vi "RX ADU.vi"(8 "error in (no error)":errorcluster, 9 "PDU_req":T1={"Function Code"=1, "Data"=[], "RTU_DataBytes"=0}, 10 "TCP connection in":refnum<k5>, 11 "MB_ADU_TCP in":refnum<class "MB_ADU_TCP.lvclass">) -> (0 "error out":errorcluster, 1 "PDU_resp":T1={"Function Code"=1, "Data"=[], "RTU_DataBytes"=0}, 2 "TCP connection out":refnum<k5>, 3 "MB_ADU_TCP out":refnum<class "MB_ADU_TCP.lvclass">)   [LabVIEW 2012, in "MB Master.lvlib" / "MB_ADU_TCP.lvclass"]
doc: "Defines the receive procedure for a Modbus TCP ADU. The received PDU is written to PDU_resp."
uses:
  MB_ADU_TCP.lvclass
  MB_PDU/MB_PDU_Cluster.ctl
  MB_ADU_TCP.lvclass/MB_ADU_TCP.ctl
  MB_ADU/MB_ADU.lvclass/MB_ADU.ctl
  MB_ADU/Read Slave ID.vi
  MB_ADU/Write RX Data.vi
  MB_ADU/Write RX Timestamp.vi
  MB Master.lvlib
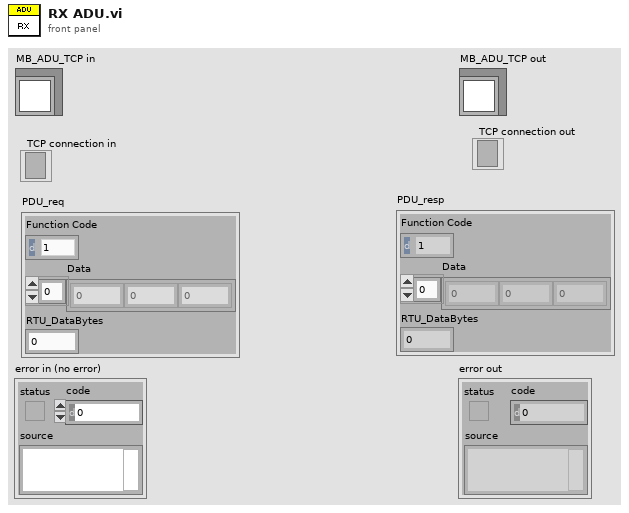
[diagram p1: front panel]
types:
  T1 = typedef "MB Master.lvlib/MB_PDU_Cluster.ctl" = cluster{"Function Code":u8, "Data":u8[], "RTU_DataBytes":i32}
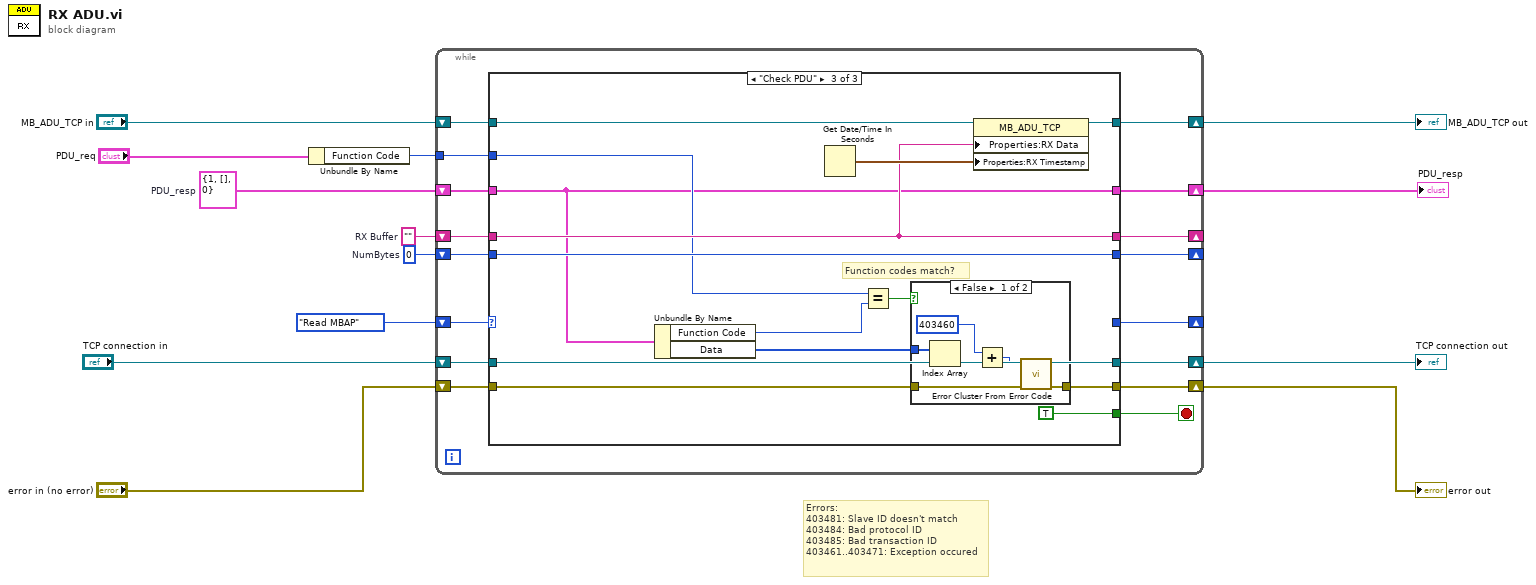
[diagram p0: block diagram]
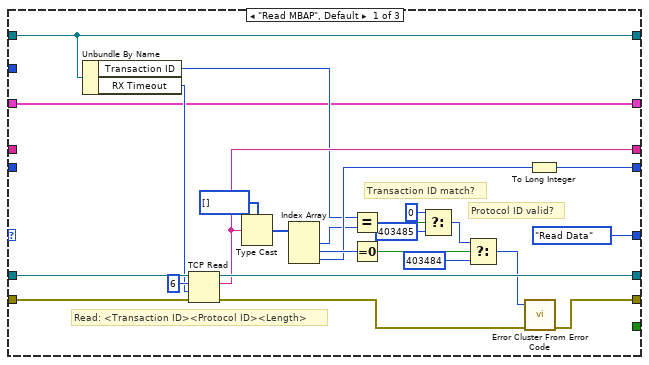
[diagram p2: hidden frame]
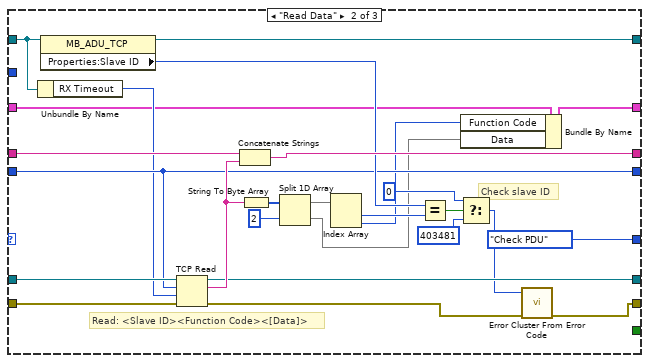
[diagram p3: hidden frame]
diagram:
  w2 = T1 {"Function Code"=1, "Data"=[], "RTU_DataBytes"=0}  # PDU_resp
  w8 = ""  # RX Buffer
  w9 = 0  # NumBytes
  # "Errors:\n403481: Slave ID doesn't match\n403484: Bad protocol ID\n403485: Bad transaction ID \n403461..403471: Exception occured"
  n1 = Unbundle By Name("PDU_req") -> ("Function Code"=w3:u8)
  n2 = while {
    shift-right: [w28] -> w13
    shift-left: "TCP connection in" -> [w29]
    shift-right: [w26] -> w10
    shift-left: "error in (no error)" -> [w25]
    shift-right: [w23] -> _
    shift-left: w9 -> [w20]
    shift-right: [w22] -> _
    shift-left: w8 -> [w21]
    shift-right: [w18] -> w5
    shift-left: "MB_ADU_TCP in" -> [w19]
    shift-right: [w17] -> _
    shift-left: enum16{"Read MBAP", "Read Data", "Check PDU"}."Read MBAP" -> [w27]
    tunnel: w3 -> [w16]
    shift-right: [w14] -> w1
    shift-left: w2 -> [w15]
    stop <- w24 stop-if-true
    n3 = case shown="\"Check PDU\"" w27 {
      tunnel: w29 -> [w41 w76 w90]
      tunnel: [w54 w77 w90] -> w28
      tunnel: [w43 w63 w86] -> w26
      tunnel: w25 -> [w51 w80 w87]
      tunnel: [_ _ TRUE ("status")] -> w24
      tunnel: [w47 w61 w91] -> w23
      tunnel: [w49 w75 w92] -> w22
      tunnel: w21 -> [_ w79 w92]
      tunnel: w20 -> [_ w61 w91]
      tunnel: w19 -> [w39 w62 w81]
      tunnel: [w39 w59 w93] -> w18
      tunnel: [enum16{"Read MBAP", "Read Data", "Check PDU"}."Read Data" enum16{"Read MBAP", "Read Data", "Check PDU"}."Check PDU" _] -> w17
      tunnel: w16 -> [_ _ w85]
      tunnel: w15 -> [w30 w58 w84]
      tunnel: [w30 w55 w84] -> w14
      frame "Read MBAP", Default {
        # "Transaction ID match?"
        # "Protocol ID valid?"
        # "Read: <Transaction ID><Protocol ID><Length>"
        n4 = Unbundle By Name(w39) -> ("Transaction ID"=w37:u16, "RX Timeout"=w31:i32)
        n5 = TCP Read(connection ID=w41, bytes to read=6, error in (no error)=w51, 9:w31) -> (connection ID out=w54:refnum<k5>, data out=w49:string, error out=w46:errorcluster)  [unwired: 1 in]
        n6 = Type Cast(type=u16[] [], x=w49) -> (*(type *) &x=w52:u16[])
        n7 = Index Array(array=w52) -> (element #1=w38:u16, element #2=w50:u16, element #3=w48:u16)  [unwired: 3 in]
        n8 = Equal?(x=w37, y=w38) -> (x = y?=w36:bool)
        n9 = Equal To 0?(x=w50) -> (x = 0?=w45:bool)
        n10 = Select(t=0, s=w36, f=403485) -> (s? t:f=w34:i32)
        n11 = Select(t=w34, s=w45, f=403484) -> (s? t:f=w42:i32)
        n12 = call <vilib>:"Error Cluster From Error Code.vi"("error in (no error)"=w46, "error code (0)"=w42) -> ("error out"=w43:errorcluster)  [unwired: 7 in]
        n13 = To Long Integer(number=w48) -> (32bit integer=w47:i32)
      }
      frame "Read Data" {
        # "Check slave ID"
        # "Read: <Slave ID><Function Code><[Data]>"
        n14 = Unbundle By Name(w62) -> ("RX Timeout"=w60:i32)
        n15 = property class="MB_ADU_TCP"(reference=w62) -> (reference out=w59:refnum<class "MB_ADU_TCP.lvclass">, "Properties:Slave ID"=w69:u8)  [unwired: 1 in, 1 out]
        n16 = TCP Read(connection ID=w76, bytes to read=w61, error in (no error)=w80, 9:w60) -> (connection ID out=w77:refnum<k5>, data out=w78:string, error out=w65:errorcluster)  [unwired: 1 in]
        n17 = Concatenate Strings(w79, w78) -> (w75:string)
        n18 = String To Byte Array(string=w78) -> (unsigned byte array=w74:u8[])
        n19 = Split 1D Array(array=w74, index=2) -> (first subarray=w73:u8[], second subarray=w56:u8[])
        n20 = Index Array(array=w73) -> (element #1=w70:u8, element #2=w57:u8)  [unwired: 2 in]
        n21 = Equal?(x=w69, y=w70) -> (x = y?=w68:bool)
        n22 = Bundle By Name(cluster=w58, "Function Code"=w57, "Data"=w56) -> (w55:T1)
        n23 = Select(t=0, s=w68, f=403481) -> (s? t:f=w64:i32)
        n24 = call <vilib>:"Error Cluster From Error Code.vi"("error in (no error)"=w65, "error code (0)"=w64) -> ("error out"=w63:errorcluster)  [unwired: 7 in]
      }
      frame "Check PDU" {
        # "Function codes match?"
        n25 = Unbundle By Name(w84) -> ("Function Code"=w83:u8, "Data"=w82:u8[])
        n26 = Get Date/Time In Seconds() -> (seconds since 1Jan1904=w94:timestamp)
        n27 = Equal?(x=w85, y=w83) -> (x = y?=w88:bool)
        n28 = case shown="False" w88 {
          tunnel: w82 -> [w99 _]
          tunnel: w87 -> [w97 w101]
          tunnel: [w96 w101] -> w86
          frame False {
            n29 = Index Array(array=w99) -> (element=w98:u8)  [unwired: 1 in]
            n30 = Add(x=403460 ("error code (0)"), y=w98) -> (x+y=w95:i32)
            n31 = call <vilib>:"Error Cluster From Error Code.vi"("error in (no error)"=w97, "error code (0)"=w95) -> ("error out"=w96:errorcluster)  [unwired: 7 in]
          }
          frame True {
          }
        }
        n32 = property class="MB_ADU_TCP"(reference=w81, "Properties:RX Data"=w92, "Properties:RX Timestamp"=w94) -> (reference out=w93:refnum<class "MB_ADU_TCP.lvclass">)  [unwired: 1 in, 1 out]
      }
    }
  }
  "error out" <- w10
  "MB_ADU_TCP out" <- w5
  "TCP connection out" <- w13
  "PDU_resp" <- w1
